vi "Digital Write Multiple Channels.vi"(7 "DAQ Module":i32, 8 "error in (no error)":errorcluster, 9 "Values":bool[](array[boolean]), 10 "Indices":i32[](array[numeric]), 11 "NI-DAQ in":refnum<class "NI-DAQ.lvclass">) -> (0 "error out":errorcluster, 3 "NI-DAQ out":refnum<class "NI-DAQ.lvclass">)   [LabVIEW 2016, in "NI-DAQ.lvclass"]
uses:
  NI-DAQ.lvclass
  NI-DAQ.lvclass/NI-DAQ.ctl
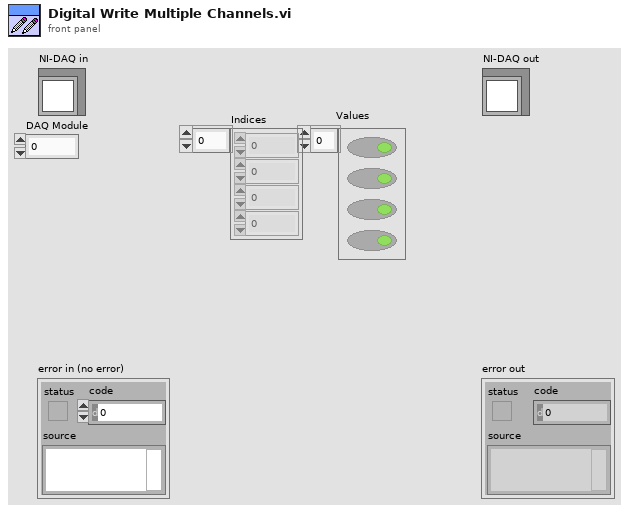
[diagram p1: front panel]
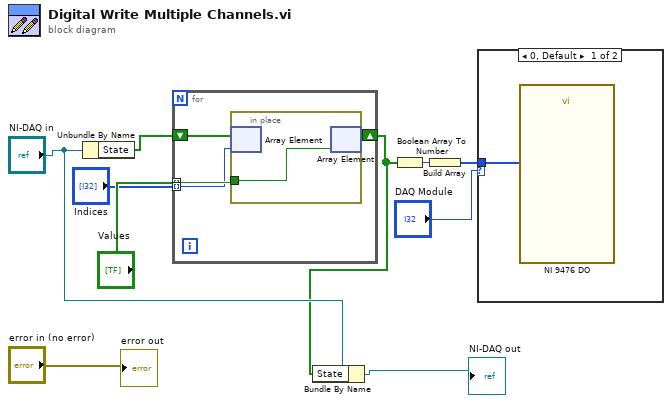
[diagram p0: block diagram]
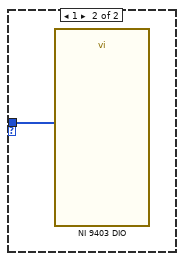
[diagram p2: hidden frame]
diagram:
  n1 = Unbundle By Name("NI-DAQ in") -> ("State"=w3:bool[])
  n2 = for {
    tunnel: "Values" -> [w14] mode=indexing
    tunnel: "Indices" -> [w13] mode=indexing
    shift-right: [w11] -> w2
    shift-left: w3 -> [w12]
    n3 = in-place {
      in-place-border: w14 -> [w15]
      n4 = in-place-array #1(w12, w13) -> ()  [unwired: 1 out]
      n5 = in-place-array #1(w15) -> (w11:bool[])  [unwired: 1 out]
    }
  }
  n6 = Bundle By Name(cluster="NI-DAQ in", "State"=w2) -> (→"NI-DAQ out":refnum<class "NI-DAQ.lvclass">)
  n7 = Boolean Array To Number(Boolean array=w2) -> (number=w9:u32)
  n8 = Build Array(w9) -> (w8:u32[])
  n9 = case shown="0, Default" "DAQ Module" {
    tunnel: w8 -> [w16 w17]
    frame 0, Default {
      n10 = call "NI 9476 DO"("data"=w16) -> ()  [unwired: 17 in, 2 out]
    }
    frame 1 {
      n11 = call "NI 9403 DIO"("data"=w17) -> ()  [unwired: 17 in, 2 out]
    }
  }
  "error out" <- "error in (no error)"
